vi "specu1a 1.0.0 Read Temperature.vi"(3 "error in (no error)":errorcluster, 5 "Device Handle":i32) -> (0 "error out":errorcluster, 1 "Temperature (°C)":dbl format="%.2f", 2 "Device Handle out":i32)   [LabVIEW 2010]
uses:
  WINDOWS/SYSTEM32/DRIVERS/specu1a.dll
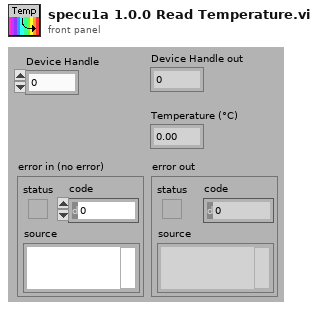
[diagram p1: front panel]
types:
  T1 = typedef "specu1a 1.0.0 Error codes.ctl" = enum16{"INVALID_HANDLE_VALUE", "USBDEV_SUCCESS", "USBDEV_INVALID_HANDLE", "USBDEV_UNSUCCESS", "USBDEV_INVALID_VALUE", "USBDEV_CHECK_NORMAL", "USBDEV_CHECK_INVALID", "USBDEV_CHECK_REMOVE", "USBDEV_CHECK_OTHER", "USBDEV_RESET_ERROR", "USBDEV_BULKSIZE_ERROR", "USBDEV_BULK_READ_ERROR", "USBDEV_BULK_NOT_UPDATED", "USBDEV_TIME_OVER_ERROR", "USBDEV_TIME_UNDER_ERROR", "USBDEV_TIME_SET_ERROR", "USBDEV_SET_GAIN_ERROR", "USBDEV_GET_TEMP_ERROR", "USBDEV_SET_TRIGGER_ERROR", "USBDEV_RW_EEP_ADDR_ERROR", "USBDEV_RW_EEP_SIZE_ERROR", "USBDEV_RW_EEP_OVER_ERROR", "USBDEV_RW_EEP_ERROR", "UNITID_PRODUCTID_CONFLICT", "UNKNOWN_ERROR"}
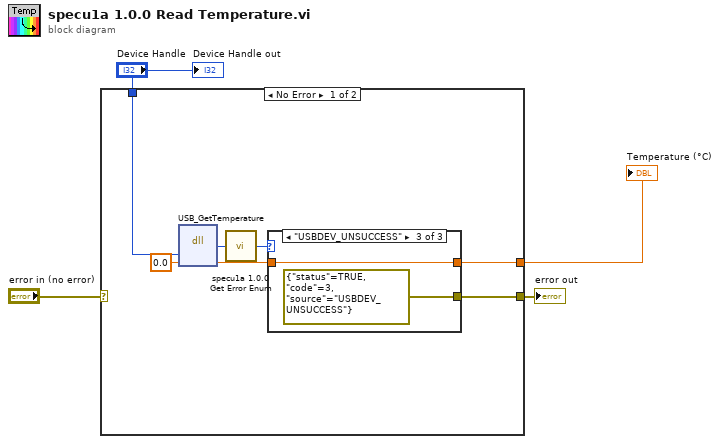
[diagram p0: block diagram]
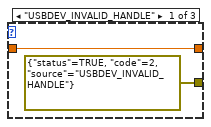
[diagram p2: hidden frame]
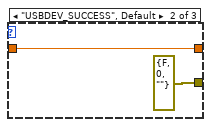
[diagram p3: hidden frame]
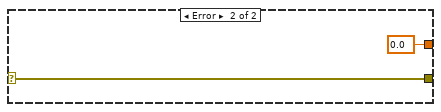
[diagram p4: hidden frame]
diagram:
  n1 = case shown="No Error" "error in (no error)" {
    selector: "error in (no error)" -> [_ w19]
    tunnel: [w10 w19] -> w3
    tunnel: [w9 0.0 ("Temperature")] -> w1
    tunnel: "Device Handle" -> [w8 _]
    frame No Error {
      n2 = dll-call lib="C:/WINDOWS/SYSTEM32/DRIVERS/specu1a.dll" fn="USB_GetTemperature" label="1.0.0 Get Temperature"("Device Handle"=w8, "Temperature"=0.0) -> (w6:u16, "Temperature"=w5:dbl)  [unwired: 4 in, 2 out]
      n3 = call "specu1a 1.0.0 Get Error Enum.vi"("Error Code in"=w6) -> ("Specu1a 1.0.0 Error code out"=w11:T1)  [unwired: 4 in]
      n4 = case shown="\"USBDEV_UNSUCCESS\"" w11 {
        tunnel: [w12 w14 w16] -> w9
        tunnel: [errorcluster {"status"=TRUE, "code"=2, "source"="USBDEV_INVALID_HANDLE"} ("error out") errorcluster {"status"=FALSE, "code"=0, "source"=""} ("error out") errorcluster {"status"=TRUE, "code"=3, "source"="USBDEV_UNSUCCESS"} ("error out")] -> w10
        tunnel: w5 -> [w12 w14 w16]
        frame "USBDEV_INVALID_HANDLE" {
        }
        frame "USBDEV_SUCCESS", Default {
        }
        frame "USBDEV_UNSUCCESS" {
        }
      }
    }
    frame Error {
    }
  }
  "error out" <- w3
  "Temperature (°C)" <- w1
  "Device Handle out" <- "Device Handle"
